vi "Scoring.vi"(0 "RisingEdge":u32, 1 "FallingEdge":u32, 2 "FallingEdge?":bool, 3 "Hit?":bool, 5 "Cluster In":T1, 6 "TargetUp?":bool) -> (7 "Cluster Out":T1, 8 "Live Score":u32, 9 "Combo":u32)   [LabVIEW 2022 SP3]
uses:
  ShargTypeDef.ctl
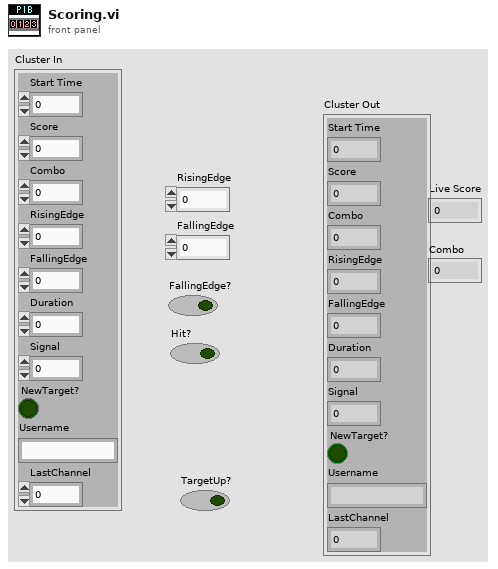
[diagram p1: front panel]
types:
  T1 = typedef "ShargTypeDef.ctl" = cluster{"Start Time":u32, "Score":u32, "Combo":u32, "RisingEdge":u32, "FallingEdge":u32, "Duration":u32, "Signal":i16, "NewTarget?":bool, "Username":string, "LastChannel":i32}
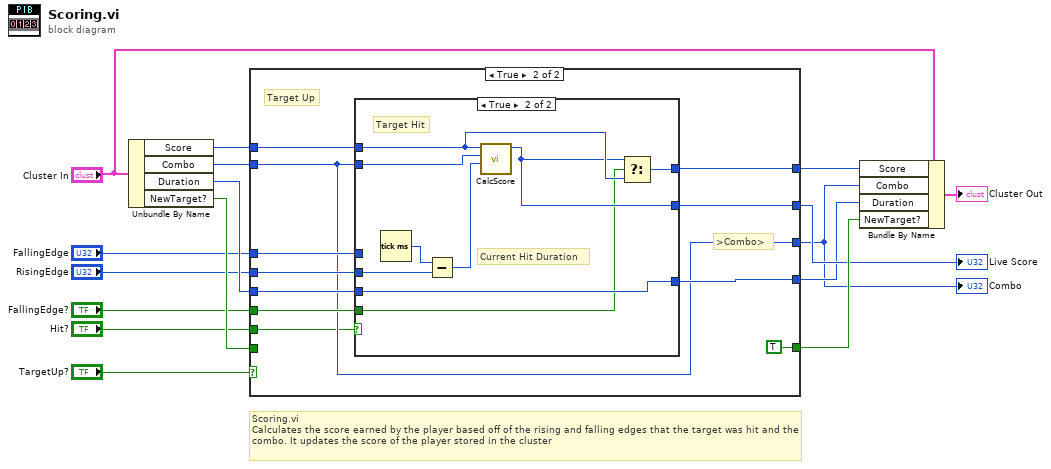
[diagram p0: block diagram]
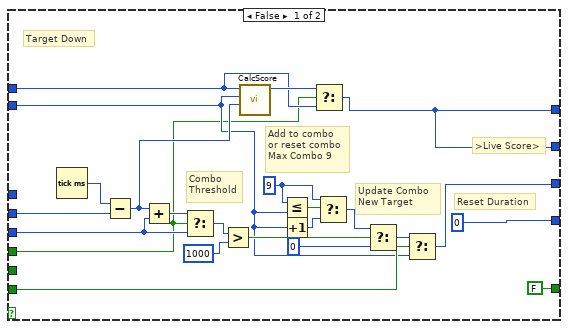
[diagram p2: hidden frame]
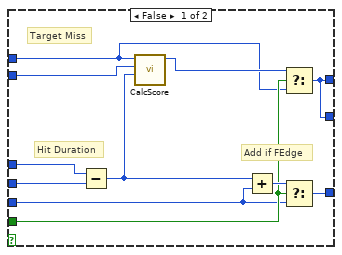
[diagram p3: hidden frame]
diagram:
  # "Scoring.vi\nCalculates the score earned by the player based off of the rising and falling edges that the target was hit and the combo. It updates the score of the player stored in the cluster"
  n1 = Unbundle By Name("Cluster In") -> ("Score"=w8:u32, "Combo"=w9:u32, "Duration"=w10:u32, "NewTarget?"=w11:bool)
  n2 = case shown="True" "TargetUp?" {
    tunnel: "Hit?" -> [_ w40]
    tunnel: "RisingEdge" -> [w31 w45]
    tunnel: "FallingEdge" -> [_ w44]
    tunnel: w10 -> [w18 w43]
    tunnel: [u32 0 ("Duration") w50] -> w14
    tunnel: "FallingEdge?" -> [w17 w49]
    tunnel: w9 -> [w25 w42]
    tunnel: [w35 w42] -> w13
    tunnel: [FALSE TRUE] -> w16
    tunnel: w11 -> [w33 _]
    tunnel: w8 -> [w21 w46]
    tunnel: [w23 w47] -> w12
    tunnel: [w23 w41] -> w15
    frame False {
      w24 = u32 9 ("t")
      # ">Live Score>"
      # "Reset Duration"
      # "Update Combo\nNew Target"
      # "Add to combo\nor reset combo\nMax Combo 9"
      # "Combo\nThreshold"
      # "Target Down"
      n3 = Tick Count (ms)() -> (millisecond timer value=w30:u32)
      n4 = Subtract(x=w30, y=w31) -> (x-y=w29:u32)
      n5 = Add(x=w29, y=w18) -> (x+y=w20:u32)
      n6 = Select(t=w20, s=w17, f=w18) -> (s? t:f=w19:u32)
      n7 = Greater?(x=w19, y=u32 1000) -> (0:w37:bool)
      n8 = call "CalcScore.vi"(">HitTime>"=w29, "Combo"=w25, "OldScore"=w21) -> ("NewScore"=w22:u32)  [unwired: 8 in]
      n9 = Less Or Equal?(x=w24, y=w25) -> (x <= y?=w26:bool)
      n10 = Increment(x=w25) -> (x+1=w27:u32)
      n11 = Select(t=w22, s=w17, f=w21) -> (s? t:f=w23:u32)
      n12 = Select(t=w24, s=w26, f=w27) -> (s? t:f=w28:u32)
      n13 = Select(t=w28, s=w37, f=u32 0) -> (s? t:f=w34:u32)
      n14 = Select(t=w34, s=w33, f=w25) -> (s? t:f=w35:u32)
    }
    frame True {
      # ">Combo>"
      # "Target Up"
      n15 = case shown="True" w40 {
        tunnel: w45 -> [w60 w69]
        tunnel: w43 -> [w55 w68]
        tunnel: w44 -> [w61 _]
        tunnel: [w57 w68] -> w50
        tunnel: w49 -> [w56 w62]
        tunnel: w46 -> [w51 w64]
        tunnel: w42 -> [w53 w66]
        tunnel: [w58 w65] -> w47
        tunnel: [w58 w63] -> w41
        frame False {
          # "Add if FEdge"
          # "Hit Duration"
          # "Target Miss"
          n16 = Subtract(x=w61, y=w60) -> (x-y=w54:u32)
          n17 = call "CalcScore.vi"(">HitTime>"=w54, "Combo"=w53, "OldScore"=w51) -> ("NewScore"=w52:u32)  [unwired: 8 in]
          n18 = Add(x=w54, y=w55) -> (x+y=w59:u32)
          n19 = Select(t=w52, s=w56, f=w51) -> (s? t:f=w58:u32)
          n20 = Select(t=w59, s=w56, f=w55) -> (s? t:f=w57:u32)
        }
        frame True {
          # "Current Hit Duration"
          # "Target Hit"
          n21 = Tick Count (ms)() -> (millisecond timer value=w70:u32)
          n22 = Subtract(x=w70, y=w69) -> (x-y=w67:u32)
          n23 = call "CalcScore.vi"(">HitTime>"=w67, "Combo"=w66, "OldScore"=w64) -> ("NewScore"=w63:u32)  [unwired: 8 in]
          n24 = Select(t=w63, s=w62, f=w64) -> (s? t:f=w65:u32)
        }
      }
    }
  }
  "Live Score" <- w15
  "Combo" <- w13
  n25 = Bundle By Name(cluster="Cluster In", "Score"=w12, "Combo"=w13, "Duration"=w14, "NewTarget?"=w16) -> (→"Cluster Out":T1)
